vi "init_theta.vi"(8 "error in (no error)":errorcluster, 10 "Commands to run":string[](array[string]), 11 "VISA Refnum in":refnum<visa-resource-name>) -> (0 "error out":errorcluster, 3 "VISA Refnum out":refnum<visa-resource-name>)   [LabVIEW 2020]
uses:
  haltnow.vi
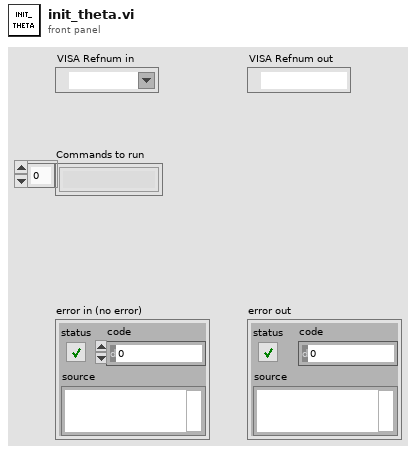
[diagram p1: front panel]
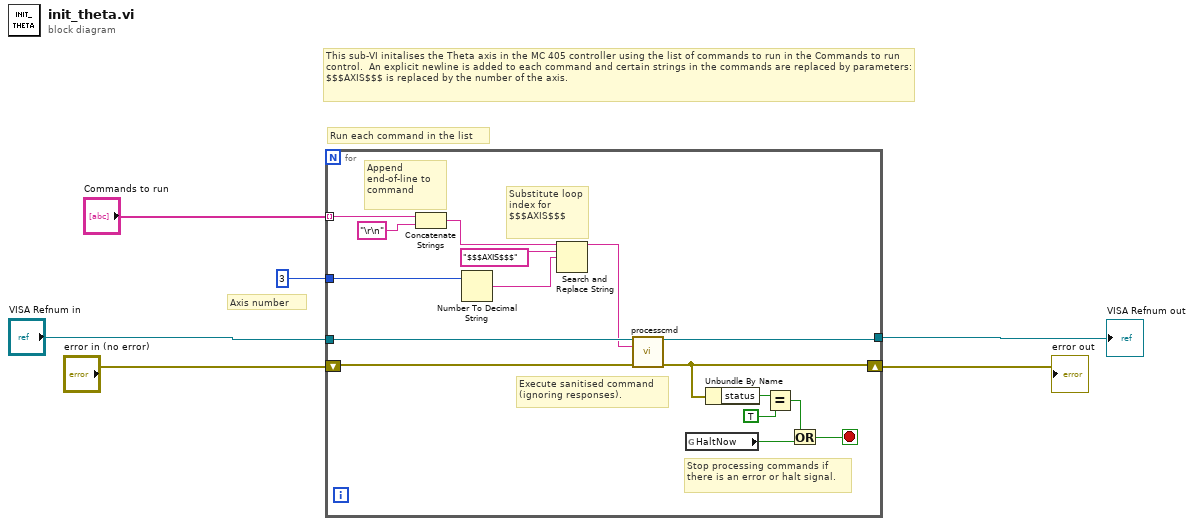
[diagram p0: block diagram]
diagram:
  # "Axis number"
  # "Run each command in the list"
  # "This sub-VI initalises the Theta axis in the MC 405 controller using the list of commands to run in the Commands to run control.  An explicit newline is added to each command and certain strings in the commands are replaced by parameters:  $$$AXIS$$$ is replaced by the number of the axis."
  n1 = for {
    shift-right: [w17] -> w3
    shift-left: "error in (no error)" -> [w22]
    tunnel: "Commands to run" -> [w18] mode=indexing
    tunnel: "VISA Refnum in" -> [w21]
    tunnel: [w20] -> w6
    tunnel: 3 -> [w8]
    stop <- w9 stop-if-true
    # "Stop processing commands if there is an error or halt signal."
    # "Execute sanitised command\n(ignoring responses)."
    # "Substitute loop index for $$$AXIS$$$"
    # "Append end-of-line to command"
    n2 = Concatenate Strings(w18, "\r\n" ("string")) -> (w13:string)
    n3 = Number To Decimal String(number=w8) -> (decimal integer string=w14:string)  [unwired: 1 in]
    n4 = Search and Replace String(input string=w13, search string="$$$AXIS$$$", replace string=w14) -> (result string=w7:string)  [unwired: 5 in, 3 out]
    n5 = call "processcmd.vi"("VISA Refnum in"=w21, "write buffer"=w7, "error in (no error)"=w22) -> ("VISA Refnum out"=w20:refnum<visa-resource-name>, "error out"=w17:errorcluster)  [unwired: 10 in, 1 out]
    n6 = global read "haltnow.vi" "HaltNow"() -> (w11:bool)
    n7 = Unbundle By Name(w17) -> ("status"=w16:bool)
    n8 = Equal?(x=w16, y=TRUE) -> (x = y?=w10:bool)
    n9 = Or(x=w10, y=w11) -> (x .or. y?=w9:bool)
  }
  "VISA Refnum out" <- w6
  "error out" <- w3
